vi "RPM Test.vi"() -> ()   [LabVIEW 2017]
uses:
  <vilib>/DAQmx/read.llb/DAQmx Read (Counter 1D DBL 1Chan NSamp).vi
  <vilib>/DAQmx/miscellaneous.llb/DAQmx Fill In Error Info.vi
  <vilib>/Analysis/NI_AALBase.lvlib
panel:
  out "Waveform Chart":dbl(graph)
  out "XY Graph":cluster{"X":dbl, "Y":dbl}[](graph)
  in  "stop":bool
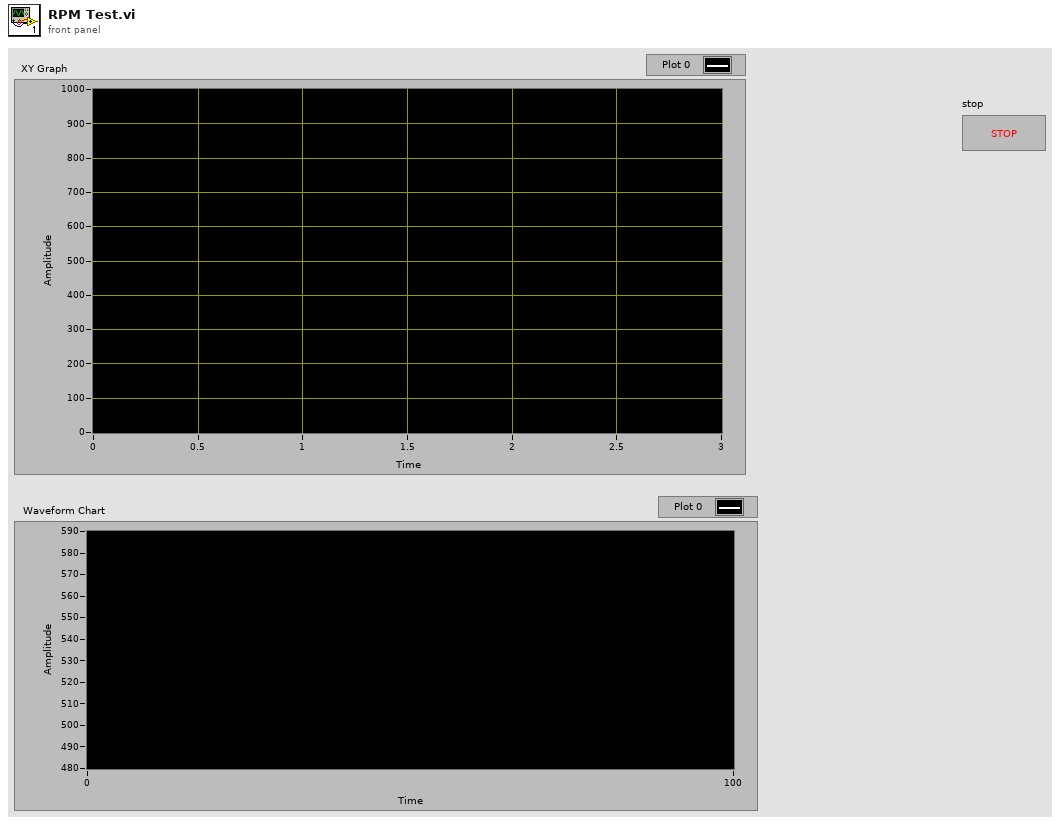
[diagram p1: front panel]
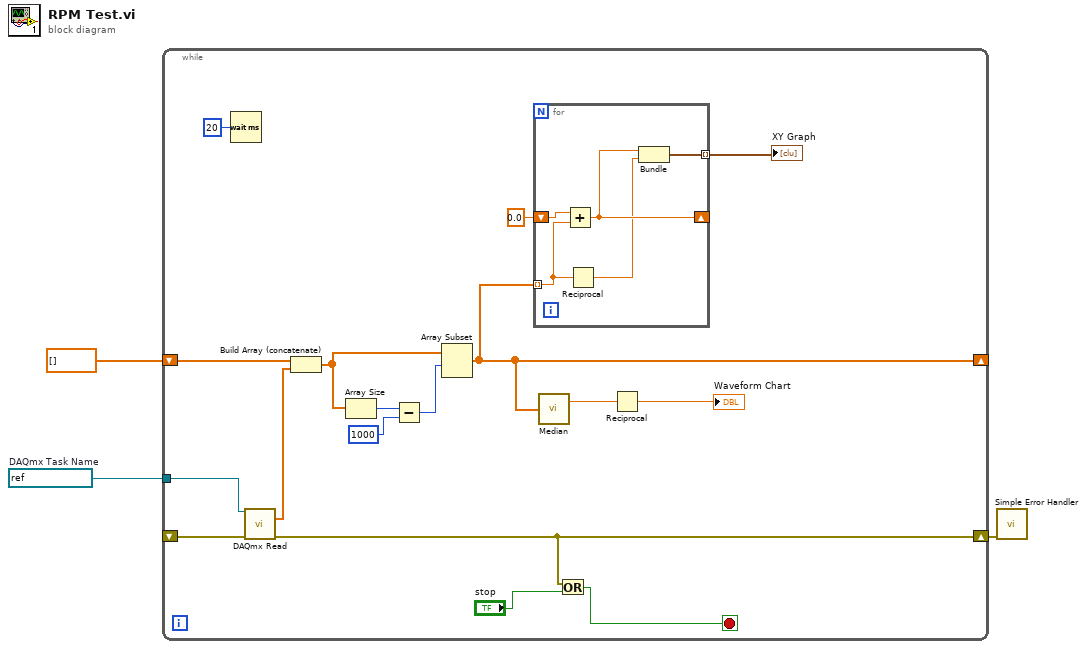
[diagram p0: block diagram]
diagram:
  w3 = refnum<k21> "PrecorCTR"  # DAQmx Task Name
  n1 = while {
    tunnel: w3 -> [w20]
    shift-right: [w15] -> w1
    shift-left: _ -> [w19]
    shift-right: [w6] -> _
    shift-left: dbl[] [] -> [w18]
    stop <- w14 stop-if-true
    n2 = Wait (ms)(milliseconds to wait=u32 20) -> ()  [unwired: 1 out]
    n3 = call-poly <vilib>:"DAQmx Read.vi"("task/channels in"=w20, "error in"=w19) -> ("data"=w17:dbl[], "error out"=w15:errorcluster)  [unwired: 11 in, 1 out]
    n4 = Build Array (concatenate)(w18, w17) -> (w10:dbl[])
    n5 = Array Size(array=w10) -> (size(s)=w13:i32)
    n6 = Subtract(x=w13, y=1000) -> (x-y=w11:i32)
    n7 = Array Subset(array=w10, index=w11) -> (w6:dbl[])  [unwired: 1 in]
    n8 = for {
      tunnel: w6 -> [w24] mode=indexing
      shift-right: [w23] -> _
      shift-left: 0.0 -> [w25]
      tunnel: [w21] -> w8 mode=indexing
      n9 = Add(x=w25, y=w24) -> (x+y=w23:dbl)
      n10 = Reciprocal(x=w24) -> (1/x=w22:dbl)
      n11 = Bundle(w23, w22) -> (w21:cluster{dbl, dbl})  [unwired: 1 in]
    }
    "XY Graph" <- w8
    n12 = call <vilib>:"Median.vi"("X"=w6) -> ("median"=w5:dbl)  [unwired: 1 out]
    n13 = Or(x=w15, y="stop") -> (x .or. y?=w14:bool)
    n14 = Reciprocal(x=w5) -> (1/x=→"Waveform Chart":dbl)
  }
  n15 = call <vilib>:"Simple Error Handler.vi"("error in (no error)"=w1) -> ()  [unwired: 4 in, 5 out]
